vi "Read Notifier.vi"(0 "LVx.lvclass in":refnum<class "LVx.lvclass">, 11 "error in (no error)":errorcluster) -> (4 "LVx.lvclass out":refnum<class "LVx.lvclass">, 6 "response notifier":T1, 15 "error out":errorcluster)   [LabVIEW 2011, in "LVx.lvlib" / "LVx.lvclass"]
uses:
  LVx.lvclass
  TypeDef/Typedef - LVx Response Notifier.ctl
  LVx.lvclass/LVx.ctl
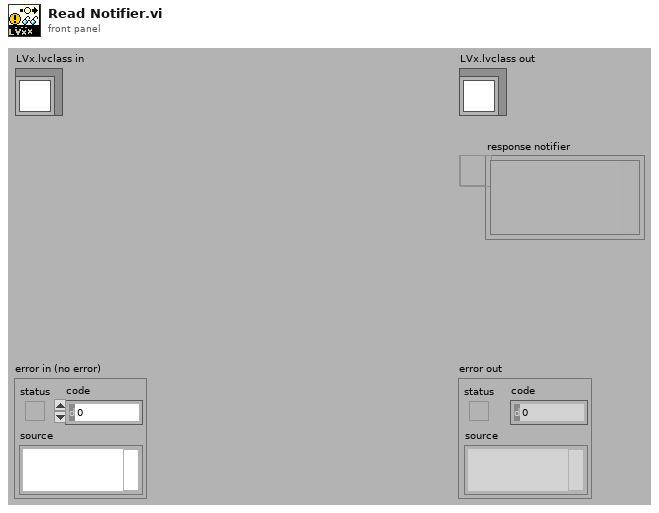
[diagram p1: front panel]
types:
  T1 = typedef "LVx.lvlib/LVx.lvclass/Typedef - LVx Response Notifier.ctl" = refnum<notifier>
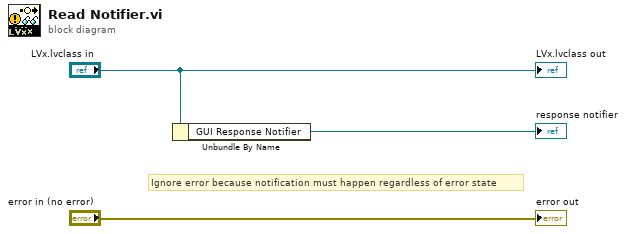
[diagram p0: block diagram]
diagram:
  # "Ignore error because notification must happen regardless of error state"
  n1 = Unbundle By Name("LVx.lvclass in") -> ("GUI Response Notifier"=→"response notifier":T1)
  "error out" <- "error in (no error)"
  "LVx.lvclass out" <- "LVx.lvclass in"
